vi "Acquire.vi"(8 "error in (no error)":errorcluster, 10 "dataRef":T1, 11 "Hardware Resources in":T2={"AI"={"DAQmx Channel"="", "Max Input"=0.0, "Min Input"=0.0, "Sample Rate"=0.0, "DAQmx Task"="", "shunt resistor location"=-1, "external shunt resistor value"=249.0}, "AO"={"DAQmx Channel"="", "Max Output"=0.0, "Min Output"=0.0, "Sample Rate"=0.0, "DAQmx Task"=""}, "DO"={"DAQmx Channel"="", "Sample Rate"=0.0, "DAQmx Task"=""}, "DI"={"DAQmx Channel"="", "Sample Rate"=0.0, "DAQmx Task"=""}, "TC"={"DAQmx Channel"="", "Max Inout"=0.0, "Min Input"=0.0, "Sample Rate"=0.0, "DAQmx Task"="", "resistance configuration"=4, "r0"=100.0, "current excitation value"=0.0025, "current excitation source"=10167, "rtd type"=12481}} {"TC"."rtd type" items=["Pt3750"=12481, "Pt3851"=10071, "Pt3911"=12482, "Pt3916"=10069, "Pt3920"=10053, "Pt3928"=12483, "Custom"=10137]; "TC"."current excitation source" items=["Internal"=10200, "External"=10167, "None"=10230]; "TC"."resistance configuration" items=["2-Wire"=2, "3-Wire"=3, "4-Wire"=4]; "AI"."shunt resistor location" items=["default"=-1, "RSE"=10083, "NRSE"=10078, "Differential"=10106, "Pseudodifferential"=12529]}) -> (0 "error out":errorcluster, 3 "Hardware Resources out":T2={"AI"={"DAQmx Channel"="", "Max Input"=0.0, "Min Input"=0.0, "Sample Rate"=0.0, "DAQmx Task"="", "shunt resistor location"=-1, "external shunt resistor value"=249.0}, "AO"={"DAQmx Channel"="", "Max Output"=0.0, "Min Output"=0.0, "Sample Rate"=0.0, "DAQmx Task"=""}, "DO"={"DAQmx Channel"="", "Sample Rate"=0.0, "DAQmx Task"=""}, "DI"={"DAQmx Channel"="", "Sample Rate"=0.0, "DAQmx Task"=""}, "TC"={"DAQmx Channel"="", "Max Inout"=0.0, "Min Input"=0.0, "Sample Rate"=0.0, "DAQmx Task"="", "resistance configuration"=4, "r0"=100.0, "current excitation value"=0.0025, "current excitation source"=10167, "rtd type"=12481}} {"TC"."rtd type" items=["Pt3750"=12481, "Pt3851"=10071, "Pt3911"=12482, "Pt3916"=10069, "Pt3920"=10053, "Pt3928"=12483, "Custom"=10137]; "TC"."current excitation source" items=["Internal"=10200, "External"=10167, "None"=10230]; "TC"."resistance configuration" items=["2-Wire"=2, "3-Wire"=3, "4-Wire"=4]; "AI"."shunt resistor location" items=["default"=-1, "RSE"=10083, "NRSE"=10078, "Differential"=10106, "Pseudodifferential"=12529]})   [LabVIEW 2024, in "Acquisition.lvlib"]
doc: "Perform the acquisition. Replace the contents of this diagram with calls to acquisition hardware."
uses:
  Acquisition.lvlib
  <vilib>/DAQmx/read.llb/DAQmx Read (Analog 2D DBL NChan NSamp).vi
  <vilib>/DAQmx/read.llb/DAQmx Read (Digital 1D Bool NChan 1Samp 1Line).vi
  <vilib>/DAQmx/read.llb/DAQmx Read (Analog 1D DBL NChan 1Samp).vi
  Hardware Configuration.ctl
  controls/dataRefs.ctl
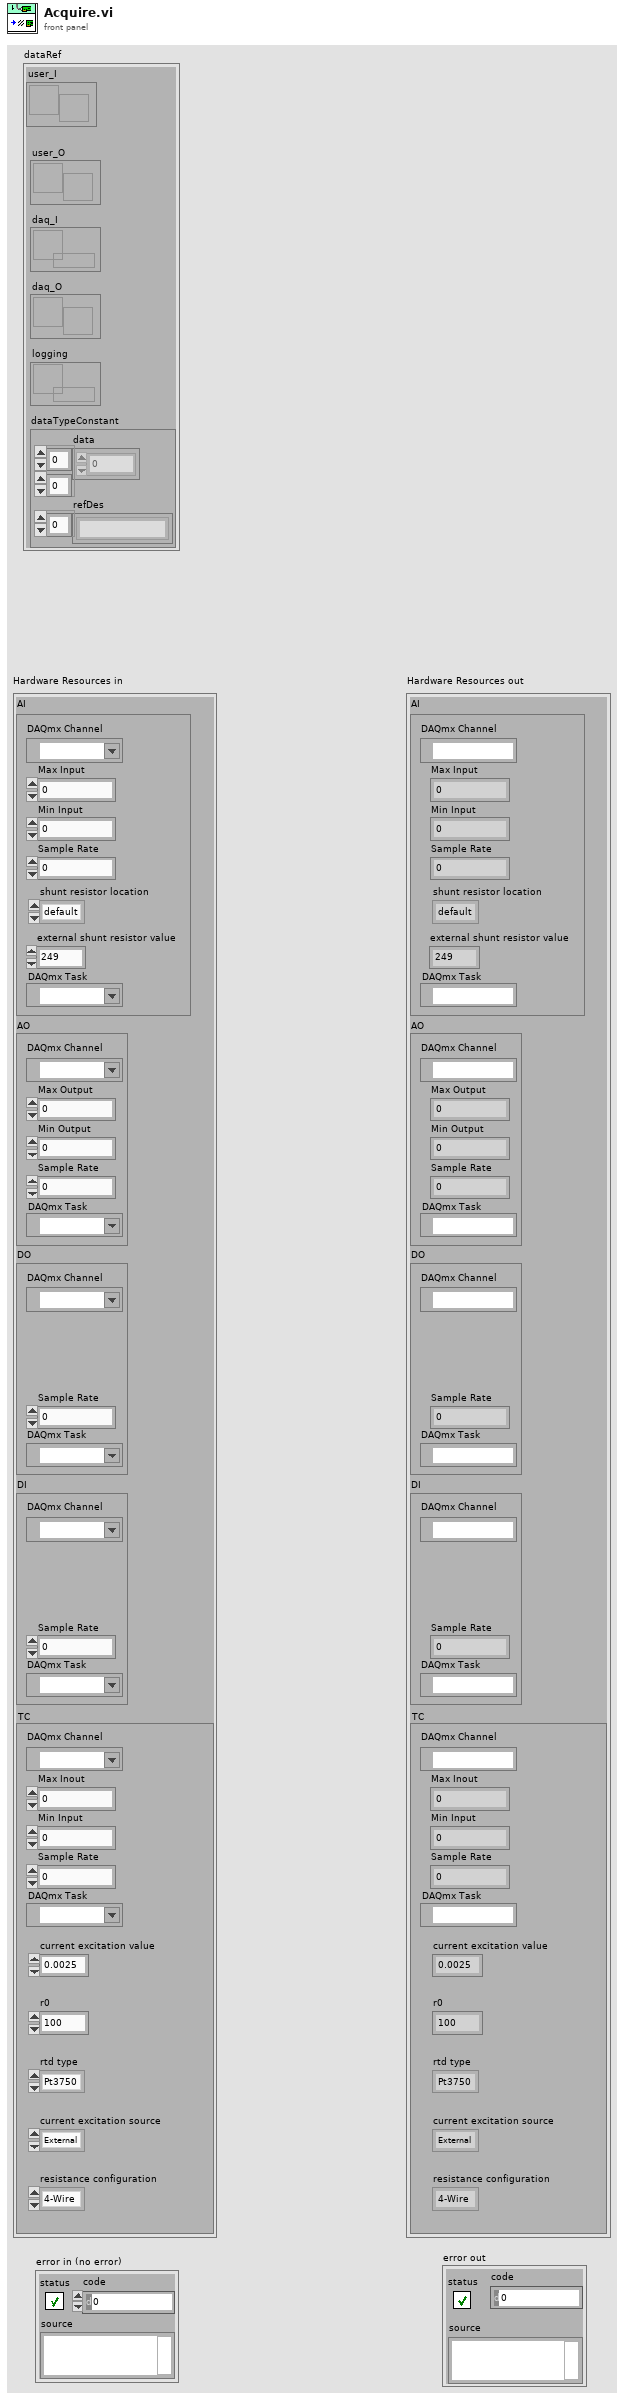
[diagram p1: front panel]
types:
  T1 = typedef "dataRefs.ctl" = cluster{"dataTypeConstant":cluster{"data":dbl[][], "refDes":string[]}, "user_I":refnum<notifier>, "user_O":refnum<notifier>, "daq_O":refnum<notifier>, "logging":refnum<queue>, "daq_I":refnum<queue>}
  T2 = typedef "Acquisition.lvlib/Hardware Configuration.ctl" = cluster{"AI":cluster{"DAQmx Channel":tag, "Max Input":dbl, "Min Input":dbl, "Sample Rate":dbl, "DAQmx Task":refnum<k21>, "shunt resistor location":i32, "external shunt resistor value":dbl}, "AO":cluster{"DAQmx Channel":tag, "Max Output":dbl, "Min Output":dbl, "Sample Rate":dbl, "DAQmx Task":refnum<k21>}, "DO":cluster{"DAQmx Channel":tag, "Sample Rate":dbl, "DAQmx Task":refnum<k21>}, "DI":cluster{"DAQmx Channel":tag, "Sample Rate":dbl, "DAQmx Task":refnum<k21>}, "TC":cluster{"DAQmx Channel":tag, "Max Inout":dbl, "Min Input":dbl, "Sample Rate":dbl, "DAQmx Task":refnum<k21>, "resistance configuration":i32, "r0":dbl, "current excitation value":dbl, "current excitation source":i32, "rtd type":i32}}
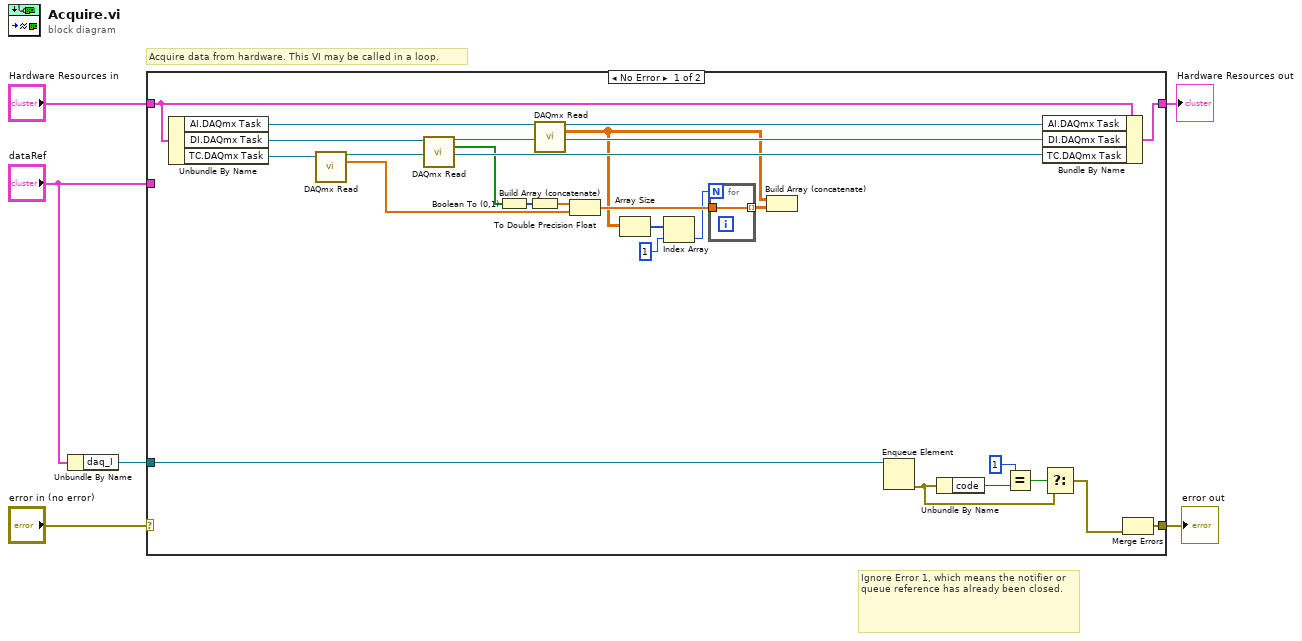
[diagram p0: block diagram]
diagram:
  # "Ignore Error 1, which means the notifier or queue reference has already been closed."
  # "Acquire data from hardware. This VI may be called in a loop."
  n1 = Unbundle By Name("dataRef") -> ("daq_I"=w1:refnum<queue>)
  n2 = case shown="No Error" "error in (no error)" {
    selector: "error in (no error)" -> [_ w33]
    tunnel: [w31 w33] -> w5
    tunnel: "Hardware Resources in" -> [w25 w34]
    tunnel: [w24 w34] -> w3
    tunnel: "dataRef" -> [_ _]
    tunnel: w1 -> [w23 _]
    frame No Error {
      n3 = Unbundle By Name(w25) -> ("AI.DAQmx Task"=w22:refnum<k21>, "DI.DAQmx Task"=w21:refnum<k21>, "TC.DAQmx Task"=w20:refnum<k21>)
      n4 = call-poly <vilib>:"DAQmx Read.vi"("task/channels in"=w20) -> ("task out"=w17:refnum<k21>, "data"=w13:dbl[])  [unwired: 12 in, 1 out]
      n5 = call-poly <vilib>:"DAQmx Read.vi"("task/channels in"=w21) -> ("task out"=w18:refnum<k21>, "data"=w16:bool[])  [unwired: 12 in, 1 out]
      n6 = Boolean To (0,1)(Boolean=w16) -> (0, 1=w15:i16[])
      n7 = To Double Precision Float(number=w15) -> (double precision float=w14:dbl[])
      n8 = call-poly <vilib>:"DAQmx Read.vi"("task/channels in"=w22) -> ("task out"=w19:refnum<k21>, "data"=w7:dbl[][])  [unwired: 12 in, 1 out]
      n9 = Build Array (concatenate)(w14, w13) -> (w10:dbl[])
      n10 = Array Size(array=w7) -> (size(s)=w12:i32[])
      n11 = Index Array(array=w12, index=1) -> (element=w9:i32)
      n12 = for {
        N: w9 -> [_]
        tunnel: w10 -> [w32]
        tunnel: [w32] -> w8 mode=indexing
      }
      n13 = Build Array (concatenate)(w7, w8) -> ()  [unwired: 1 out]
      n14 = Enqueue Element(queue=w23) -> (error out=w30:errorcluster)  [unwired: 3 in, 2 out]
      n15 = Unbundle By Name(w30) -> ("code"=w27:i32)
      n16 = Equal?(x=1, y=w27) -> (x = y?=w29:bool)
      n17 = Bundle By Name(cluster=w25, "AI.DAQmx Task"=w19, "DI.DAQmx Task"=w18, "TC.DAQmx Task"=w17) -> (w24:T2)
      n18 = Select(s=w29, f=w30) -> (s? t:f=w26:errorcluster)  [unwired: 1 in]
      n19 = Merge Errors(w26) -> (w31:errorcluster)  [unwired: 1 in]
    }
    frame Error {
    }
  }
  "Hardware Resources out" <- w3
  "error out" <- w5
